vi "Sequence Check Timeout.vi"(11 "Sequencer Data Context IN":T1={"Sequencer State"=enum."Clear Drive Fault", "Event Timeout"=-1, "Current Index"=0, "Duration (Seconds)"=0.0, "Turbine RPM"=0.0, "Pump RPM"=0.0, "Sequence Timeout"=0}) -> (0 "error out":errorcluster, 3 "Sequencer Data Context OUT":T1={"Sequencer State"=enum."Clear Drive Fault", "Event Timeout"=-1, "Current Index"=0, "Duration (Seconds)"=0.0, "Turbine RPM"=0.0, "Pump RPM"=0.0, "Sequence Timeout"=0})   [LabVIEW 2024, in "Auto Modo.lvlib"]
uses:
  Auto Modo.lvlib
  Sequencer Data Context.ctl
  Sequencer State.ctl
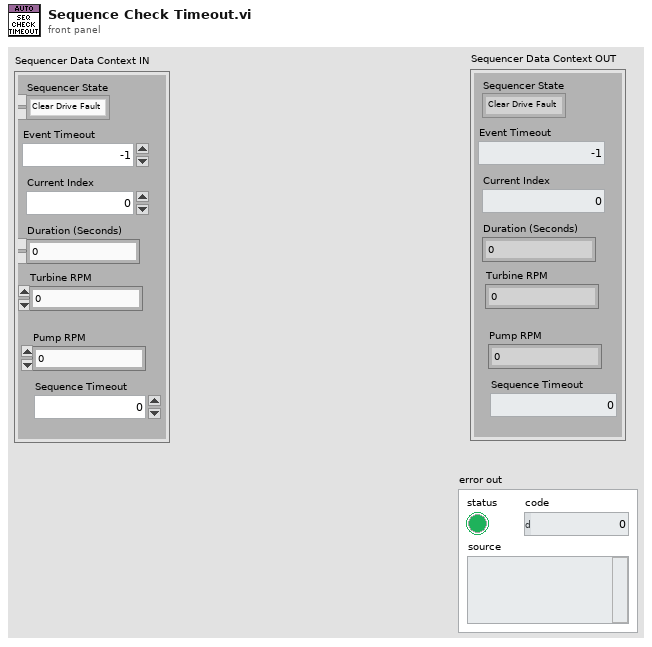
[diagram p1: front panel]
types:
  T1 = typedef "Auto Modo.lvlib/Sequencer Data Context.ctl" = cluster{"Sequencer State":T2, "Event Timeout":i32, "Current Index":i32, "Duration (Seconds)":dbl, "Turbine RPM":dbl, "Pump RPM":dbl, "Sequence Timeout":i32}
  T2 = typedef "Auto Modo.lvlib/Sequencer State.ctl" = enum16{"Clear Drive Fault", "Check Drive Fault", "Set Ready to Switch ON", "Final"}
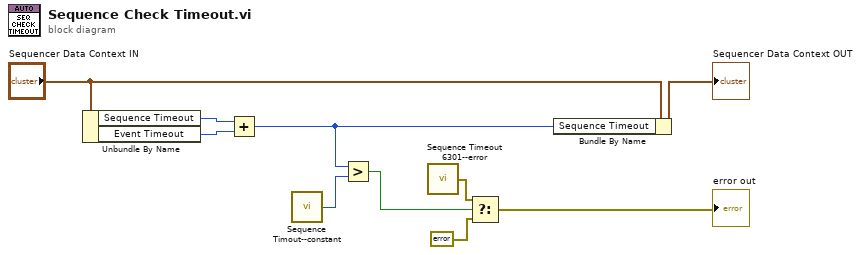
[diagram p0: block diagram]
diagram:
  n1 = Unbundle By Name("Sequencer Data Context IN") -> ("Sequence Timeout"=w8:i32, "Event Timeout"=w9:i32)
  n2 = Add(x=w8, y=w9) -> (x+y=w6:i32)
  n3 = call "Sequence Timout--constant.vi"() -> ("Sequence Timeout (ms)"=w5:i32)  [unwired: 1 in]
  n4 = Greater?(x=w6, y=w5) -> (0:w4:bool)
  n5 = call "Sequence Timeout 6301--error.vi"() -> ("error out"=w2:errorcluster)  [unwired: 1 in]
  n6 = Select(t=w2, s=w4, f=errorcluster {"status"=FALSE, "code"=0, "source"=""} ("error constant")) -> (s? t:f=→"error out":errorcluster)
  n7 = Bundle By Name(cluster="Sequencer Data Context IN", "Sequence Timeout"=w6) -> (→"Sequencer Data Context OUT":T1)
